vi "close.vi"(8 "error in (no error)":errorcluster, 11 "SalProcess in":refnum<class "SalProcess.lvclass">) -> (0 "error out":errorcluster, 3 "SalProcess out":refnum<class "SalProcess.lvclass">)   [LabVIEW 2018, in "SalProcess.lvclass"]
doc: "Close the internal references."
uses:
  SalProcess.lvclass
  SalProcess.lvclass/SalProcess.ctl
  LibReader/LibReader.lvclass
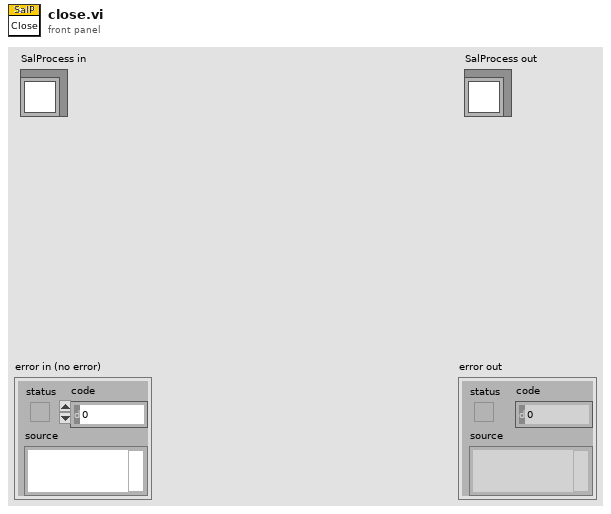
[diagram p1: front panel]
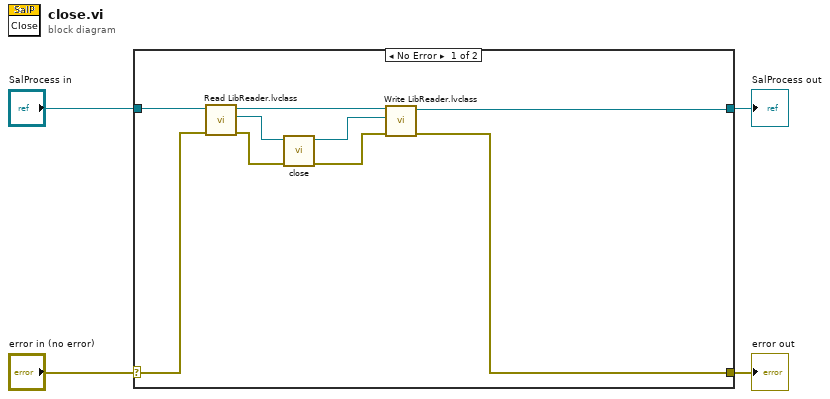
[diagram p0: block diagram]
diagram:
  n1 = case shown="No Error" "error in (no error)" {
    selector: "error in (no error)" -> [w12 w15]
    tunnel: [w5 w15] -> w3
    tunnel: [w8 w14] -> w1
    tunnel: "SalProcess in" -> [w13 w14]
    frame No Error {
      n2 = call "Read LibReader.lvclass.vi"("error in (no error)"=w12, "SalProcess in"=w13) -> ("error out"=w10:errorcluster, "LibReader.lvclass"=w11:refnum<class "LibReader.lvclass">, "SalProcess out"=w9:refnum<class "SalProcess.lvclass">)  [unwired: 7 in]
      n3 = call "close.vi"("error in (no error)"=w10, "LibReader in"=w11) -> ("error out"=w6:errorcluster, "LibReader out"=w7:refnum<class "LibReader.lvclass">)  [unwired: 8 in]
      n4 = call "Write LibReader.lvclass.vi"("error in (no error)"=w6, "LibReader.lvclass"=w7, "SalProcess in"=w9) -> ("error out"=w5:errorcluster, "SalProcess out"=w8:refnum<class "SalProcess.lvclass">)  [unwired: 7 in]
    }
    frame Error {
    }
  }
  "error out" <- w3
  "SalProcess out" <- w1
